vi "tm_initialize.vi"(8 "error in (no error)":errorcluster {"code" format="%.0x"}) -> (0 "error out":errorcluster {"code" format="%.0x"}, 3 "Number Of Cameras":u32)   [LabVIEW 2012]
uses:
  tmcamcon.dll
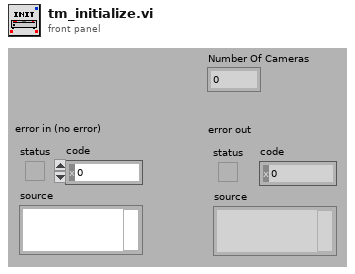
[diagram p1: front panel]
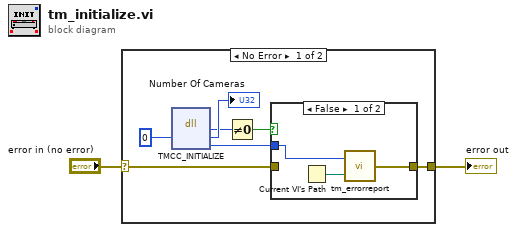
[diagram p0: block diagram]
diagram:
  n1 = case shown="No Error" "error in (no error)" {
    selector: "error in (no error)" -> [w7 w14]
    tunnel: [w6 w14] -> w1
    frame No Error {
      n2 = dll-call lib="tmcamcon.dll" fn="TMCC_INITIALIZE"("Count"=u32 0) -> ("return type"=w3:u32, "Count"=→"Number Of Cameras":u32, "Erval"=w9:i32)  [unwired: 4 in, 2 out]
      n3 = Not Equal To 0?(x=w3) -> (x != 0?=w4:bool)
      n4 = case shown="False" w4 {
        tunnel: w7 -> [_ w13]
        tunnel: [w12 w13] -> w6
        tunnel: w9 -> [w10 _]
        frame False {
          n5 = Current VI's Path() -> (path=w11:path)
          n6 = call <userlib>:"tm_errorreport.vi"("Source"=w11, "Error"=w10) -> ("error out"=w12:errorcluster)
        }
        frame True {
        }
      }
    }
    frame Error {
    }
  }
  "error out" <- w1
